vi "Read Convex Hull Image.vi"(8 "error in (no error)":errorcluster, 11 "Video Cam Processor in":refnum<class "Video Cam Processor.lvclass">) -> (0 "error out":errorcluster, 2 "Image":T1, 3 "Video Cam Processor out":refnum<class "Video Cam Processor.lvclass">)   [LabVIEW 2018, in "Video Cam Processor.lvclass"]
uses:
  Video Cam Processor.lvclass
  C:/Users/aaron.jencks/Documents/GitHub/emerson_seed_object_detection/LabVIEW/Projects/Paul's Video Viewer/Classes/Video File/Video File.lvclass
  <vilib>/vision/Image Controls.llb/IMAQ Image.ctl
  Video Cam Processor.lvclass/Video Cam Processor.ctl
  f6caba72-c6ea-4ae3-be71-7210b2fcc362.vi
  Video File/Video File.lvclass
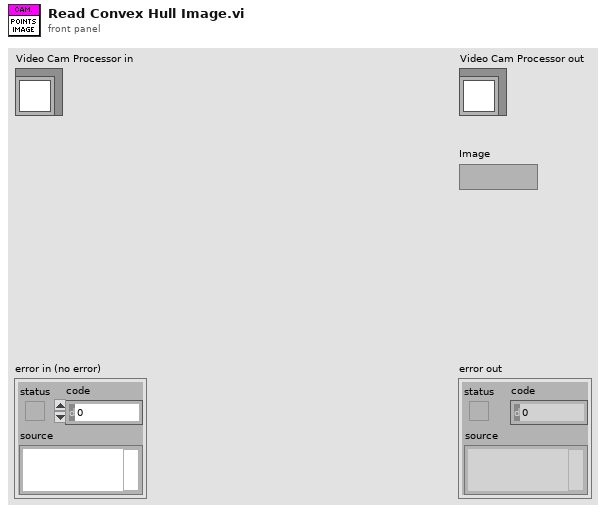
[diagram p1: front panel]
types:
  T1 = typedef "IMAQ Image.ctl" = refnum<image>
  T2 = typedef "Image Type" = u32
  T3 = typedef "Video Cam Processor.lvclass/Hull Point STYP.ctl" = cluster{"X":i32, "Y":i32}
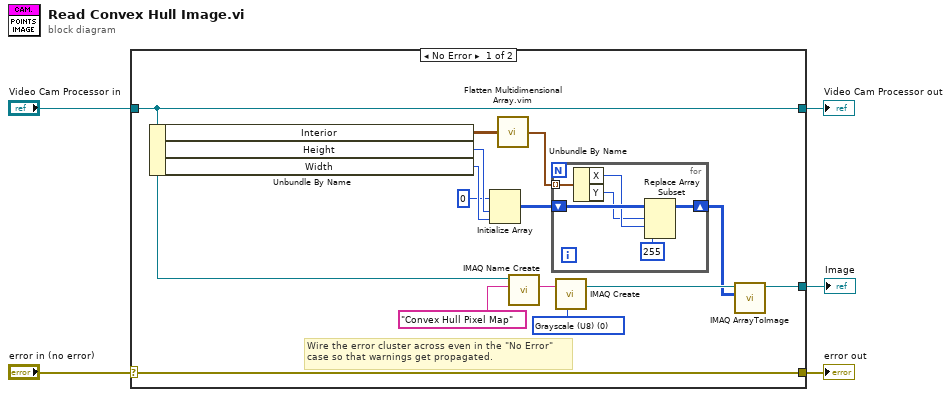
[diagram p0: block diagram]
diagram:
  n1 = case shown="No Error" "error in (no error)" {
    selector: "error in (no error)" -> [w19 w27]
    tunnel: [w19 w27] -> w4
    tunnel: [w15 w26] -> w2
    tunnel: "Video Cam Processor in" -> [w15 w26]
    tunnel: [w6 _] -> w1
    frame No Error {
      w12 = T2 0 items=["Grayscale (U8)", "Grayscale (I16)", "Grayscale (SGL)", "Complex (CSG)", "RGB (U32)", "HSL (U32)", "RGB (U64)", "Grayscale (U16)"] ("Image Type")
      # "Wire the error cluster across even in the \"No Error\"\ncase so that warnings get propagated."
      n2 = Unbundle By Name(w15) -> ("Interior"=w10:T3[][], "Height"=w18:i32, "Width"=w17:i32)
      n3 = Initialize Array(u8 0 ("element"), w18, w17) -> (w11:u8[][])
      n4 = call "Flatten Multidimensional Array.vim"("Array"=w10) -> ("output array"=w9:T3[])  [unwired: 14 in]
      n5 = call "IMAQ Name Create.vi"("Name (\"\")"="Convex Hull Pixel Map" ("Name (\"\")"), "Video File in"=w15) -> ("Name Out"=w13:string)  [unwired: 7 in, 2 out]
      n6 = for {
        tunnel: w9 -> [w24] mode=indexing
        shift-right: [w20] -> w7
        shift-left: w11 -> [w25]
        n7 = Unbundle By Name(w24) -> ("X"=w23:i32, "Y"=w22:i32)
        n8 = Replace Array Subset(array=w25, new element=u8 255 ("new element/subarray"), index (row)=w22, index (col)=w23) -> (w20:u8[][])
      }
      n9 = call "IMAQ Create"("Image Name"=w13, "Image Type"=w12) -> ("New Image"=w8:T1)  [unwired: 3 in, 1 out]
      n10 = call "IMAQ ArrayToImage"("Image Pixels (U8)"=w7, "Image"=w8) -> ("Image Out"=w6:T1)  [unwired: 8 in, 1 out]
    }
    frame Error {
    }
  }
  "error out" <- w4
  "Video Cam Processor out" <- w2
  "Image" <- w1
